vi "Configure Measurement Edge.vi"   [LabVIEW 2016, in "Agilent 2000 3000 X-Series.lvlib"]
doc: "Configures the measurement edge."
uses:
  Agilent 2000 3000 X-Series.lvlib
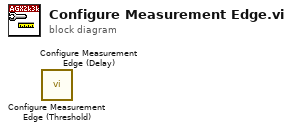
[diagram p0: block diagram]
diagram:
  n1 = call "Configure Measurement Edge (Threshold).vi"() -> ()  [unwired: 10 in, 2 out]
  n2 = call "Configure Measurement Edge (Delay).vi"() -> ()  [unwired: 10 in, 2 out]
